vi "Slit Controller.vi"(8 "error in (no error)":errorcluster, 10 "Notifiers":T1, 11 "All Message Queue Cluster":T2) -> (0 "error out":errorcluster)   [LabVIEW 2013]
uses:
  Lib QMH/AllMessageQueue Cluster.ctl
  Lib QMH/Message Cluster.ctl
  Lib Notifier/Notifier.ctl
  Lib QMH/MessageQueues.lvlib
  Lib Log/Logging.lvlib
  Lib Notifier/Notifier.lvlib
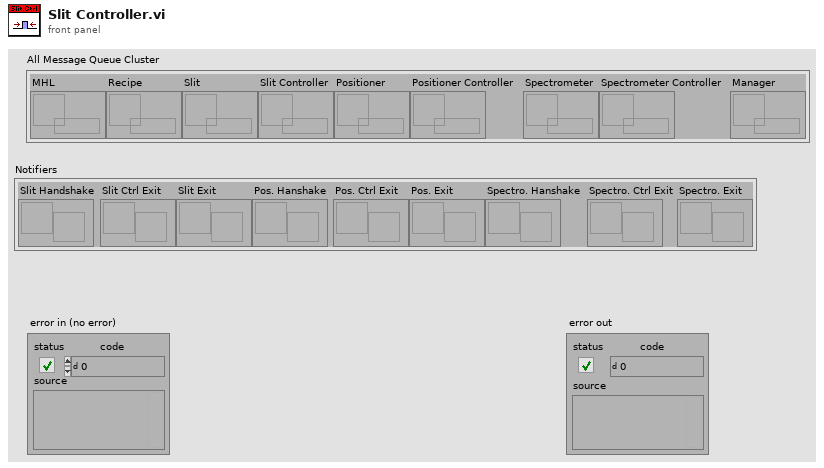
[diagram p1: front panel]
types:
  T1 = typedef "Notifier.lvlib/Notifier.ctl" = cluster{"Slit Handshake":refnum<notifier>, "Slit Ctrl Exit":refnum<notifier>, "Slit Exit":refnum<notifier>, "Pos. Hanshake":refnum<notifier>, "Pos. Ctrl Exit":refnum<notifier>, "Pos. Exit":refnum<notifier>, "Spectro. Hanshake":refnum<notifier>, "Spectro. Ctrl Exit":refnum<notifier>, "Spectro. Exit":refnum<notifier>}
  T2 = typedef "MessageQueues.lvlib/AllMessageQueue Cluster.ctl" = cluster{"MHL":refnum<queue>, "Recipe":refnum<queue>, "Slit":refnum<queue>, "Slit Controller":refnum<queue>, "Positioner":refnum<queue>, "Positioner Controller":refnum<queue>, "Spectrometer":refnum<queue>, "Spectrometer Controller":refnum<queue>, "Manager":refnum<queue>}
  T3 = enum16{"open", "replace", "create", "open or create", "replace or create", "replace or create with confirmation"}
  T4 = cluster{"état":bool, "code":i32, "source":string}
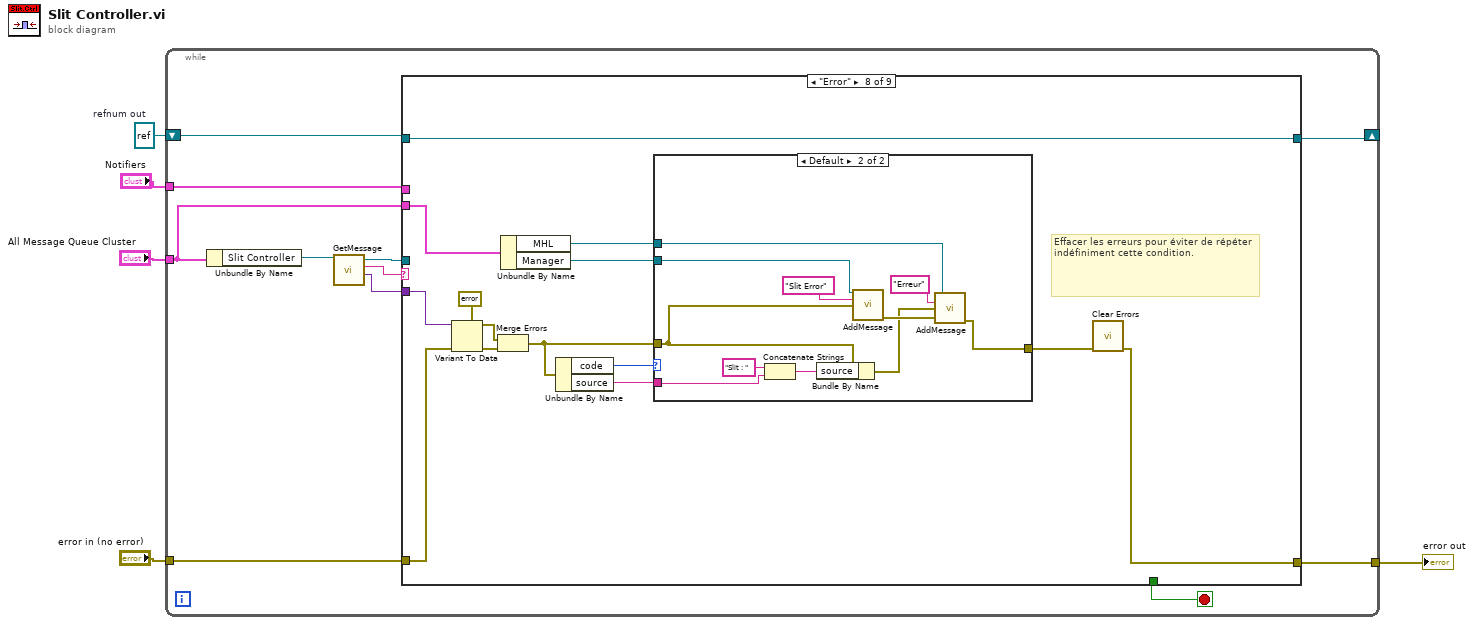
[diagram p0: block diagram]
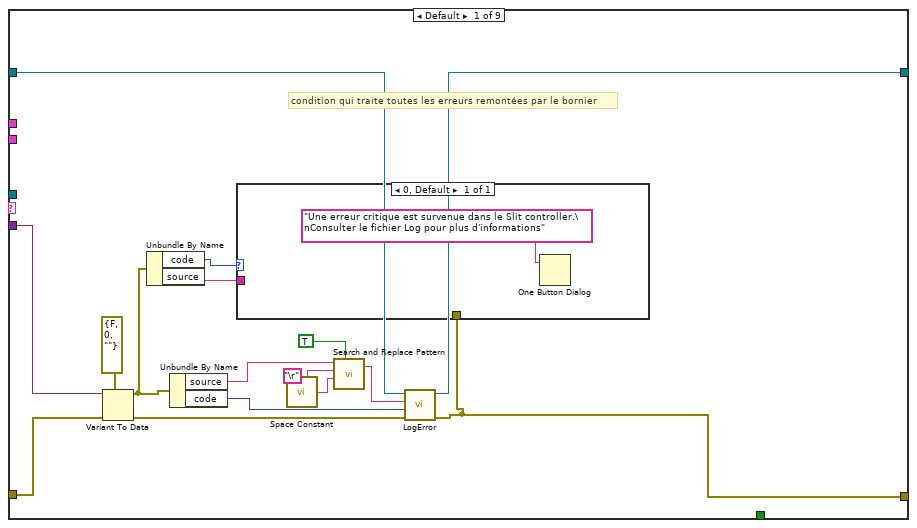
[diagram p2: hidden frame]
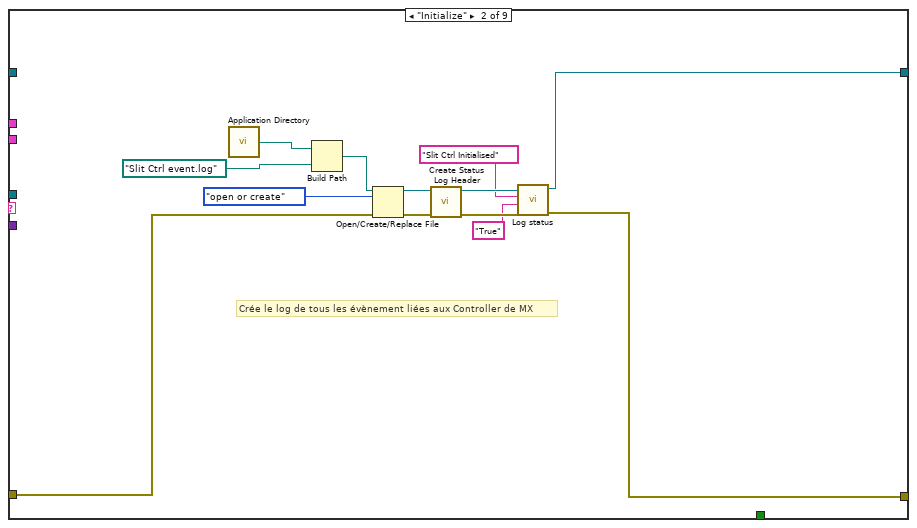
[diagram p3: hidden frame]
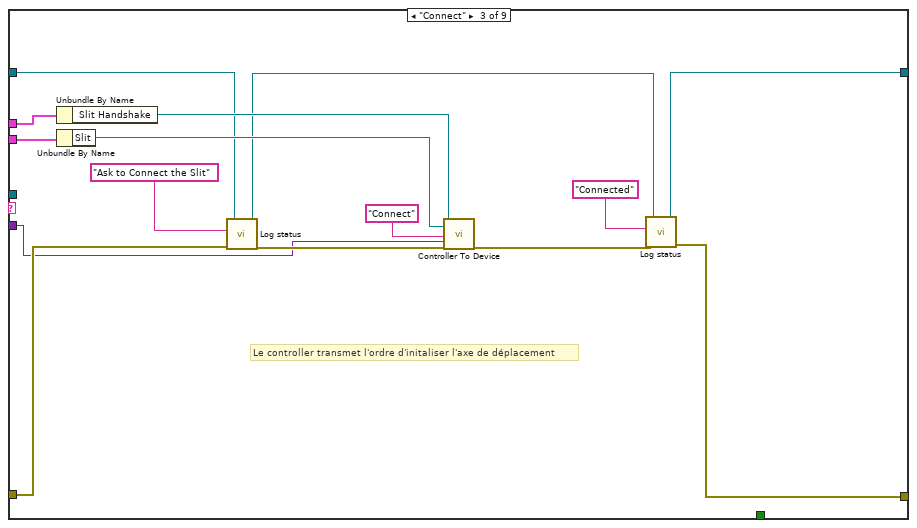
[diagram p4: hidden frame]
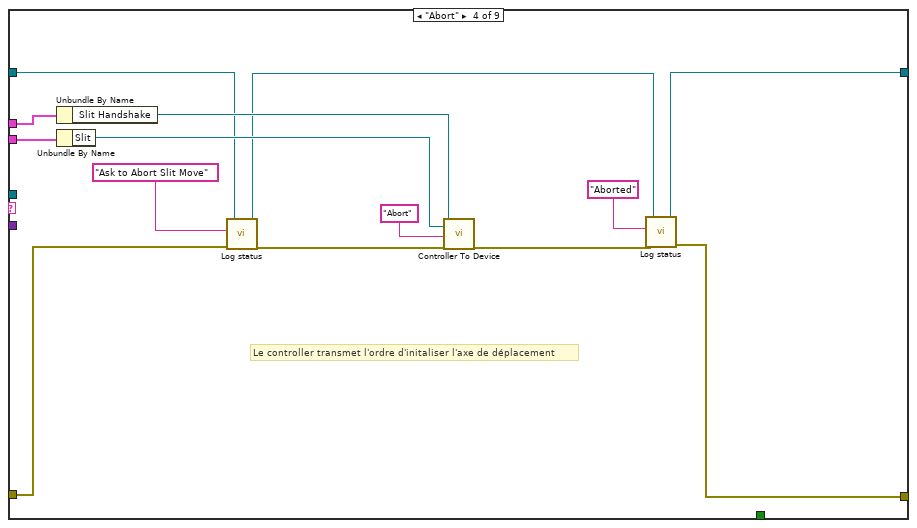
[diagram p5: hidden frame]
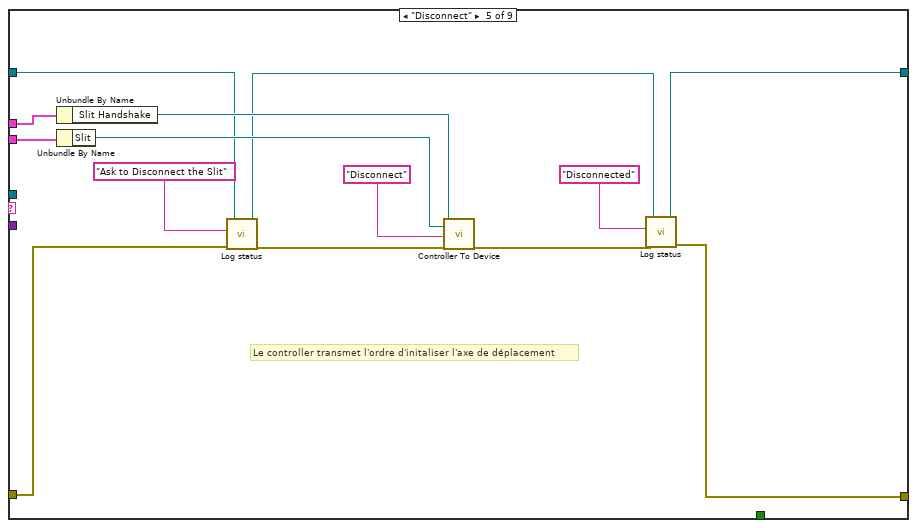
[diagram p6: hidden frame]
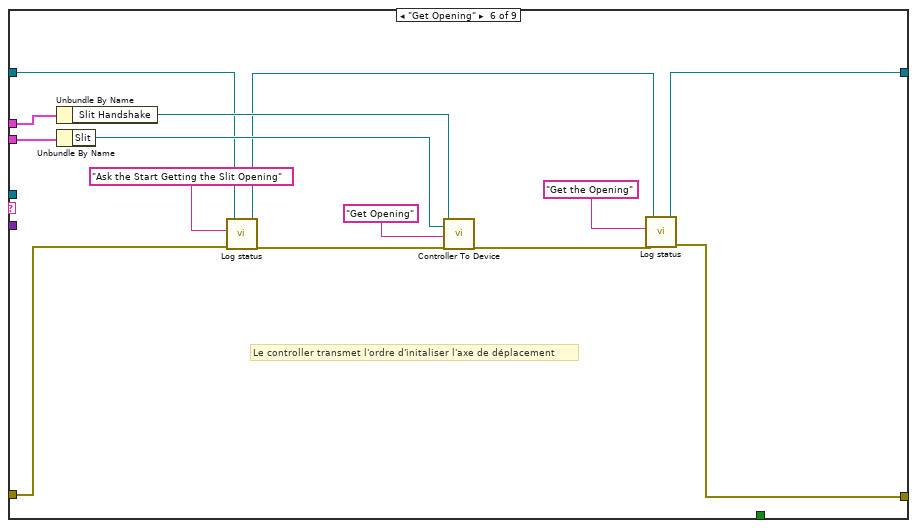
[diagram p7: hidden frame]
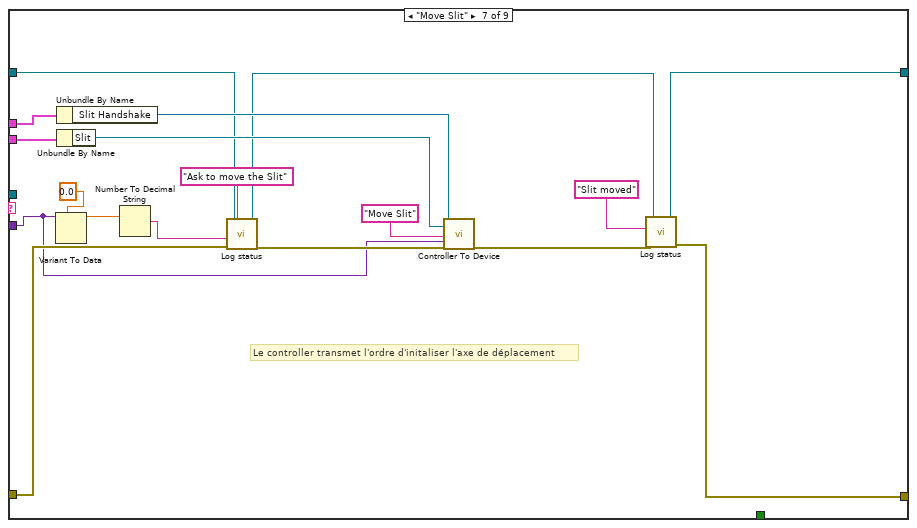
[diagram p8: hidden frame]
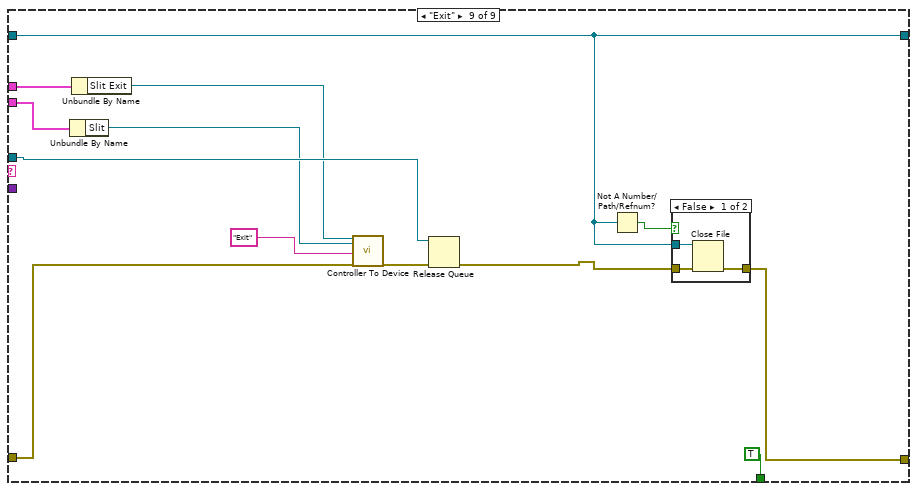
[diagram p10: hidden frame]
diagram:
  w2 = refnum<file> refnum  # refnum out
  n1 = while {
    tunnel: "All Message Queue Cluster" -> [w10]
    tunnel: "Notifiers" -> [w9]
    tunnel: "error in (no error)" -> [w8]
    tunnel: [w15] -> w1
    shift-right: [w12] -> _
    shift-left: w2 -> [w13]
    stop <- w14 stop-if-true
    n2 = Unbundle By Name(w10) -> ("Slit Controller"=w16:refnum<queue>)
    n3 = call "GetMessage.vi"("Message queue"=w16) -> ("Data"=w7:variant, "Message"=w6:string, "Dup Message Queue"=w11:refnum<queue>)  [unwired: 7 in, 1 out]
    n4 = case shown="\"Error\"" w6 {
      tunnel: w9 -> [_ _ w61 w75 w89 w103 w121 _ w157]
      tunnel: w10 -> [_ _ w60 w74 w88 w102 w120 w124 w156]
      tunnel: w8 -> [w21 w36 w49 w63 w77 w91 w109 w126 w152]
      tunnel: [_ _ _ _ _ _ _ _ TRUE] -> w14
      tunnel: w11 -> [_ _ _ _ _ _ _ _ w158]
      tunnel: w7 -> [w19 _ w47 _ _ _ w104 w127 _]
      tunnel: [w17 w34 w52 w66 w80 w94 w112 w135 w154] -> w12
      tunnel: w13 -> [w18 _ w56 w70 w84 w98 w116 w135 w154]
      tunnel: [w20 w35 w54 w68 w82 w96 w114 w125 w155] -> w15
      frame Default {
        # "condition qui traite toutes les erreurs remontées par le bornier"
        n5 = Variant To Data(error in=w21, type=errorcluster {"status"=FALSE, "code"=0, "source"=""} ("error in (no error)"), Variant=w19) -> (data=w32:errorcluster, error out=w23:errorcluster)
        n6 = Unbundle By Name(w32) -> ("code"=w30:i32, "source"=w31:string)
        n7 = Unbundle By Name(w32) -> ("source"=w25:string, "code"=w24:i32)
        n8 = call <vilib>:"Space Constant.vi"() -> ("String"=w27:string)
        n9 = call <vilib>:"Search and Replace Pattern.vi"("string"=w25, "regular expression (\"\")"="\r", "replace string (\"\")"=w27, "replace all? (F)"=TRUE) -> ("result string"=w28:string)  [unwired: 1 in, 1 out]
        n10 = call "LogError.vi"("entrée d'erreur"=w23, "Code"=w24, "Source"=w28, "Error log refnum In"=w18) -> ("error out"=w20:errorcluster, "Error log refnum out"=w17:refnum<file>)  [unwired: 6 in]
        n11 = case shown="0, Default" w30 {
          tunnel: w31 -> [_]
          tunnel: w20 -> [_]
          frame 0, Default {
            n12 = One Button Dialog(message="Une erreur critique est survenue dans le Slit controller.\nConsulter le fichier Log pour plus d'informations" ("chaîne de format")) -> ()  [unwired: 1 in, 1 out]
          }
        }
      }
      frame "Initialize" {
        # "Crée le log de tous les évènement liées aux Controller de MX"
        n13 = call <vilib>:"Application Directory.vi"() -> ("Application Directory"=w43:path)
        n14 = Build Path(base path=w43, name or relative path=path "Slit Ctrl event.log") -> (appended path=w45:path)
        n15 = Open/Create/Replace File(file path (use dialog)=w45, error in=w36, operation (0:open)=T3."open or create" ("opération (0 : open)")) -> (refnum out=w41:refnum<file>, error out=w42:errorcluster)  [unwired: 3 in, 1 out]
        n16 = call "Create Status Log Header.vi"("entrée d'erreur"=w42, "Log File Refnum In"=w41) -> ("sortie d'erreur"=w40:errorcluster, "Log File Refnum out"=w39:refnum<file>)  [unwired: 8 in]
        n17 = call "Log status.vi"("entrée d'erreur"=w40, "Event Data String (-)"="True", "Event string"="Slit Ctrl Initialised", "Log File Refnum In"=w39) -> ("error out"=w35:errorcluster, "Log File Refnum out"=w34:refnum<file>)  [unwired: 6 in]
      }
      frame "Connect" {
        # "Le controller transmet l'ordre d'initaliser l'axe de déplacement"
        n18 = Unbundle By Name(w61) -> ("Slit Handshake"=w59:refnum<notifier>)
        n19 = Unbundle By Name(w60) -> ("Slit"=w58:refnum<queue>)
        n20 = call "Log status.vi"("entrée d'erreur"=w49, "Event string"="Ask to Connect the Slit", "Log File Refnum In"=w56) -> ("error out"=w57:errorcluster, "Log File Refnum out"=w53:refnum<file>)  [unwired: 7 in]
        n21 = call "Controller To Device.vi"("Notifier"=w59, "Message queue"=w58, "Message"="Connect", "Data"=w47, "entrée d'erreur"=w57) -> ("sortie d'erreur"=w55:errorcluster)  [unwired: 12 in, 2 out]
        n22 = call "Log status.vi"("entrée d'erreur"=w55, "Event string"="Connected", "Log File Refnum In"=w53) -> ("error out"=w54:errorcluster, "Log File Refnum out"=w52:refnum<file>)  [unwired: 7 in]
      }
      frame "Abort" {
        # "Le controller transmet l'ordre d'initaliser l'axe de déplacement"
        n23 = Unbundle By Name(w75) -> ("Slit Handshake"=w73:refnum<notifier>)
        n24 = Unbundle By Name(w74) -> ("Slit"=w72:refnum<queue>)
        n25 = call "Log status.vi"("entrée d'erreur"=w63, "Event string"="Ask to Abort Slit Move", "Log File Refnum In"=w70) -> ("error out"=w71:errorcluster, "Log File Refnum out"=w67:refnum<file>)  [unwired: 7 in]
        n26 = call "Controller To Device.vi"("Notifier"=w73, "Message queue"=w72, "Message"="Abort", "entrée d'erreur"=w71) -> ("sortie d'erreur"=w69:errorcluster)  [unwired: 13 in, 2 out]
        n27 = call "Log status.vi"("entrée d'erreur"=w69, "Event string"="Aborted", "Log File Refnum In"=w67) -> ("error out"=w68:errorcluster, "Log File Refnum out"=w66:refnum<file>)  [unwired: 7 in]
      }
      frame "Disconnect" {
        # "Le controller transmet l'ordre d'initaliser l'axe de déplacement"
        n28 = Unbundle By Name(w89) -> ("Slit Handshake"=w87:refnum<notifier>)
        n29 = Unbundle By Name(w88) -> ("Slit"=w86:refnum<queue>)
        n30 = call "Log status.vi"("entrée d'erreur"=w77, "Event string"="Ask to Disconnect the Slit", "Log File Refnum In"=w84) -> ("error out"=w85:errorcluster, "Log File Refnum out"=w81:refnum<file>)  [unwired: 7 in]
        n31 = call "Controller To Device.vi"("Notifier"=w87, "Message queue"=w86, "Message"="Disconnect", "entrée d'erreur"=w85) -> ("sortie d'erreur"=w83:errorcluster)  [unwired: 13 in, 2 out]
        n32 = call "Log status.vi"("entrée d'erreur"=w83, "Event string"="Disconnected", "Log File Refnum In"=w81) -> ("error out"=w82:errorcluster, "Log File Refnum out"=w80:refnum<file>)  [unwired: 7 in]
      }
      frame "Get Opening" {
        # "Le controller transmet l'ordre d'initaliser l'axe de déplacement"
        n33 = Unbundle By Name(w103) -> ("Slit Handshake"=w101:refnum<notifier>)
        n34 = Unbundle By Name(w102) -> ("Slit"=w100:refnum<queue>)
        n35 = call "Log status.vi"("entrée d'erreur"=w91, "Event string"="Ask the Start Getting the Slit Opening", "Log File Refnum In"=w98) -> ("error out"=w99:errorcluster, "Log File Refnum out"=w95:refnum<file>)  [unwired: 7 in]
        n36 = call "Controller To Device.vi"("Notifier"=w101, "Message queue"=w100, "Message"="Get Opening", "entrée d'erreur"=w99) -> ("sortie d'erreur"=w97:errorcluster)  [unwired: 13 in, 2 out]
        n37 = call "Log status.vi"("entrée d'erreur"=w97, "Event string"="Get the Opening", "Log File Refnum In"=w95) -> ("error out"=w96:errorcluster, "Log File Refnum out"=w94:refnum<file>)  [unwired: 7 in]
      }
      frame "Move Slit" {
        # "Le controller transmet l'ordre d'initaliser l'axe de déplacement"
        n38 = Variant To Data(type=0.0, Variant=w104) -> (data=w106:dbl)  [unwired: 1 in, 1 out]
        n39 = Unbundle By Name(w121) -> ("Slit Handshake"=w119:refnum<notifier>)
        n40 = Unbundle By Name(w120) -> ("Slit"=w118:refnum<queue>)
        n41 = Number To Decimal String(number=w106) -> (decimal integer string=w105:string)  [unwired: 1 in]
        n42 = call "Log status.vi"("entrée d'erreur"=w109, "Event Data String (-)"=w105, "Event string"="Ask to move the Slit", "Log File Refnum In"=w116) -> ("error out"=w117:errorcluster, "Log File Refnum out"=w113:refnum<file>)  [unwired: 6 in]
        n43 = call "Controller To Device.vi"("Notifier"=w119, "Message queue"=w118, "Message"="Move Slit", "Data"=w104, "entrée d'erreur"=w117) -> ("sortie d'erreur"=w115:errorcluster)  [unwired: 12 in, 2 out]
        n44 = call "Log status.vi"("entrée d'erreur"=w115, "Event string"="Slit moved", "Log File Refnum In"=w113) -> ("error out"=w114:errorcluster, "Log File Refnum out"=w112:refnum<file>)  [unwired: 7 in]
      }
      frame "Error" {
        # "Effacer les erreurs pour éviter de répéter indéfiniment cette condition."
        n45 = Variant To Data(error in=w126, type=T4 {"état"=FALSE, "code"=0, "source"=""} ("sortie d'erreur"), Variant=w127) -> (data=w132:T4, error out=w133:errorcluster)
        n46 = Merge Errors(w132, w133) -> (w129:errorcluster)
        n47 = Unbundle By Name(w124) -> ("MHL"=w123:refnum<queue>, "Manager"=w128:refnum<queue>)
        n48 = Unbundle By Name(w129) -> ("code"=w130:i32, "source"=w122:string)
        n49 = case shown="Default" w130 {
          tunnel: [w136 w145] -> w131
          tunnel: w129 -> [w136 w138]
          tunnel: w128 -> [_ w142]
          tunnel: w123 -> [_ w143]
          tunnel: w122 -> [_ w139]
          frame 5000..5002 {
          }
          frame Default {
            n50 = Concatenate Strings("Slit : " ("string"), w139) -> (w140:string)
            n51 = Bundle By Name(cluster=w138, "source"=w140) -> (w137:errorcluster)
            n52 = call "AddMessage.vi"("Message queue"=w142, "Message"="Slit Error", "Data"=w138) -> ("error out"=w144:errorcluster)  [unwired: 11 in, 1 out]
            n53 = call "AddMessage.vi"("Message queue"=w143, "Message"="Erreur", "Data"=w137, "entrée d'erreur (pas d'erreur)"=w144) -> ("error out"=w145:errorcluster)  [unwired: 10 in, 1 out]
          }
        }
        n54 = call <vilib>:"Clear Errors.vi"("error in (no error)"=w131) -> ("error out"=w125:errorcluster)  [unwired: 6 in]
      }
      frame "Exit" {
        n55 = Unbundle By Name(w156) -> ("Slit"=w149:refnum<queue>)
        n56 = Unbundle By Name(w157) -> ("Slit Exit"=w150:refnum<notifier>)
        n57 = call "Controller To Device.vi"("Notifier"=w150, "Message queue"=w149, "Message"="Exit", "entrée d'erreur"=w152) -> ("sortie d'erreur"=w153:errorcluster)  [unwired: 13 in, 2 out]
        n58 = Release Queue(queue=w158, error in (no error)=w153) -> (error out=w148:errorcluster)  [unwired: 1 in, 2 out]
        n59 = Not A Number/Path/Refnum?(number/path/refnum=w154) -> (NaN/Path/Refnum?=w159:bool)
        n60 = case shown="False" w159 {
          tunnel: [w163 w164] -> w155
          tunnel: w148 -> [w162 w164]
          tunnel: w154 -> [w161 _]
          frame False {
            n61 = Close File(refnum=w161, error in=w162) -> (error out=w163:errorcluster)  [unwired: 1 out]
          }
          frame True {
          }
        }
      }
    }
  }
  "error out" <- w1
